vi "Spectrum.vi"(0 "Bins":u32=500, 2 "Gain":dbl=1.0, 3 "Remove Polynomial Order":i32=2, 4 "Waveform 1":cluster{dbl, dbl, dbl[]}, 5 "Binning":bool) -> (1 "Cluster":T1)   [LabVIEW 2020]
uses:
  <vilib>/Analysis/4window.llb/windowTd.ctl
  <vilib>/measure/maspectr.llb/Power Spectrum and PSD Export Mode.ctl
  <instrlib>/tio-labview/Labview Signal Processing/Log Range.vi
  <vilib>/measure/maspectr.llb/FFT Power Spectrum and PSD for 1 Chan.vi
  <vilib>/measure/NI_MAPro.lvlib
  <vilib>/Analysis/NI_AALPro.lvlib
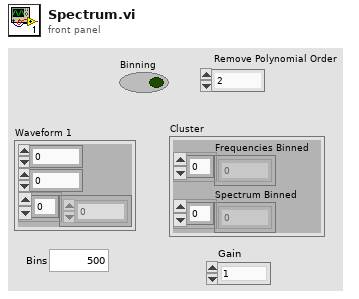
[diagram p1: front panel]
types:
  T1 = cluster{"Frequencies Binned":dbl[], "Spectrum Binned":dbl[]}
  T2 = typedef "NI_MAPro.lvlib/Power Spectrum and PSD Export Mode.ctl" = u16
  T3 = typedef "NI_AALPro.lvlib/windowTd.ctl" = u32
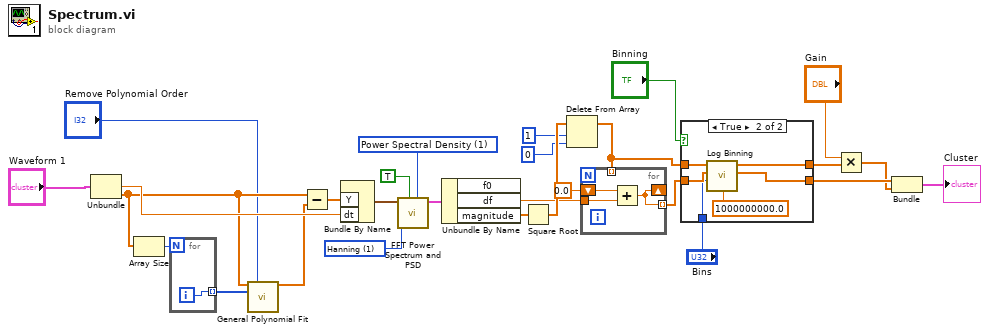
[diagram p0: block diagram]
diagram:
  w20 = T2 1 items=["Power Spectrum", "Power Spectral Density"] ("export mode")
  w17 = T3 1 items=["Rectangle"=0, "Hanning"=1, "Hamming"=2, "Blackman-Harris"=3, "Exact Blackman"=4, "Blackman"=5, "Flat Top"=6, "4 Term B-Harris "=7, "7 Term B-Harris"=8, "Low Sidelobe"=9, "Blackman Nuttall"=11, "Triangle"=30, "Bartlett-Hanning"=31, "Bohman"=32, "Parzen"=33, "Welch"=34, "Kaiser"=60, "Dolph-Chebyshev"=61, "Gaussian"=62] ("window")
  n1 = Unbundle("Waveform 1") -> (w10:dbl, w7:dbl[])  [unwired: 1 out]
  n2 = Array Size(array=w7) -> (size(s)=w9:i32)
  n3 = for {
    N: w9 -> [_]
    tunnel: [w29] -> w8 mode=indexing
    i -> [w29]
  }
  n4 = call <vilib>:"General Polynomial Fit.vi"("Y"=w7, "polynomial order"="Remove Polynomial Order", "X"=w8) -> ("Best Polynomial Fit"=w6:dbl[])  [unwired: 9 in, 3 out]
  n5 = Subtract(x=w7, y=w6) -> (x-y=w14:dbl[])
  n6 = Bundle By Name("Y"=w14, "dt"=w10) -> (w22:waveform(dbl))  [unwired: 1 in]
  n7 = call-poly <vilib>:"FFT Power Spectrum and PSD.vi"("export mode"=w20, "restart averaging (F)"=TRUE, "window"=w17, "time signal"=w22) -> ("Power Spectrum / PSD"=w15:cluster{"f0":dbl, "df":dbl, "magnitude":dbl[]})  [unwired: 4 in, 3 out]
  n8 = Unbundle By Name(w15) -> ("df"=w16:dbl, "magnitude"=w21:dbl[])  [unwired: 1 out]
  n9 = Square Root(x=w21) -> (sqrt(x)=w26:dbl[])
  n10 = Delete From Array(array=w26, length=1, index=0) -> (array with subset deleted=w27:dbl[])  [unwired: 1 out]
  n11 = for {
    tunnel: w16 -> [w32]
    shift-right: [w30] -> _
    shift-left: 0.0 -> [w31]
    tunnel: [w30] -> w19 mode=indexing
    tunnel: w27 -> [_] mode=indexing
    n12 = Add(x=w31, y=w32) -> (x+y=w30:dbl)
  }
  n13 = case shown="True" "Binning" {
    tunnel: [w33 w40] -> w13
    tunnel: w19 -> [w33 w39]
    tunnel: [w34 w38] -> w4
    tunnel: w27 -> [w34 w37]
    tunnel: "Bins" -> [_ w35]
    frame False {
    }
    frame True {
      n14 = call <instrlib>:"Log Binning.vi"("Max Freq"=dbl[unit] 1000000000.0, "Number Elements"=w35, "Frequencies"=w39, "Spectrum"=w37) -> ("Frequencies Binned"=w40:dbl[], "Spectrum Binned"=w38:dbl[])  [unwired: 2 in]
    }
  }
  n15 = Multiply(x="Gain", y=w4) -> (x*y=w3:dbl[])
  n16 = Bundle("Frequencies Binned"=w13, w3) -> (→"Cluster":cluster{"Frequencies Binned":dbl[], dbl[]})  [unwired: 1 out]
